vi "Flatten.vi"(8 "error in":errorcluster, 9 "Data":T1) -> (0 "error out":errorcluster, 2 "Buffer":u8[](array[numeric]) format="%.0x")   [LabVIEW 2020, in "Error.lvlib"]
uses:
  Error.lvlib
  Data.ctl
  lv-protoc/LV-Proto/LV-Proto.lvlib
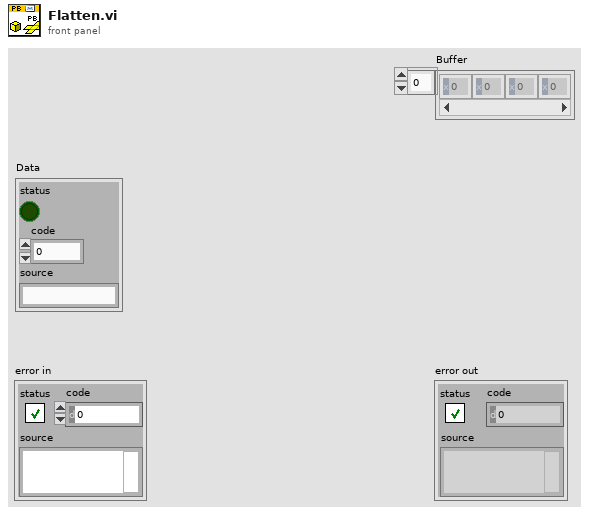
[diagram p1: front panel]
types:
  T1 = typedef "Error.lvlib/Data.ctl" = errorcluster
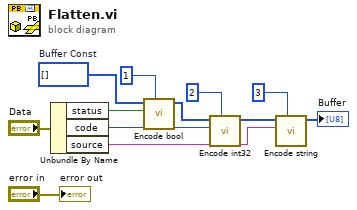
[diagram p0: block diagram]
diagram:
  w10 = u8[] []  # Buffer Const
  n1 = Unbundle By Name("Data") -> ("status"=w8:bool, "code"=w5:i32, "source"=w2:string)
  n2 = call "Encode bool.vi"("Field Number"=1, "Bool"=w8, "Buffer in"=w10) -> ("Buffer"=w7:u8[])  [unwired: 8 in]
  n3 = call "Encode int32.vi"("Field Number"=2, "int32"=w5, "Buffer in"=w7) -> ("Buffer"=w4:u8[])  [unwired: 8 in]
  n4 = call "Encode string.vi"("Field Number"=3, "string"=w2, "Buffer in"=w4) -> ("Buffer"=→"Buffer":u8[])  [unwired: 8 in]
  "error out" <- "error in"
